vi "Build Help.vi"(8 "Error In":errorcluster) -> (0 "Error Out":errorcluster, 3 "stdout":string)   [LabVIEW 2017, in "Scripts.lvlib"]
uses:
  Scripts.lvlib
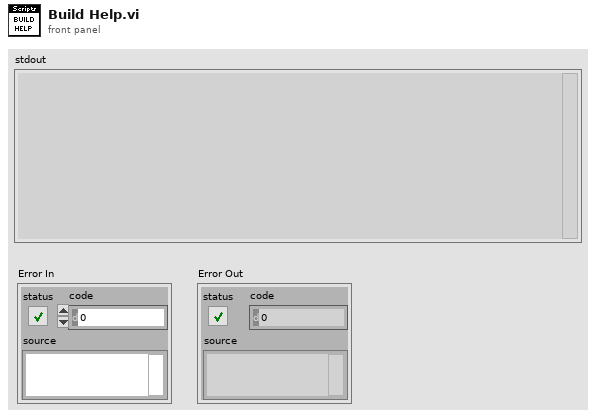
[diagram p1: front panel]
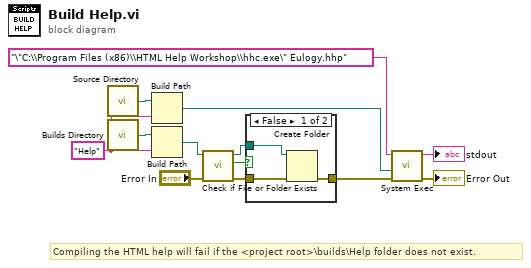
[diagram p0: block diagram]
diagram:
  w7 = "Help" ("name or relative path")
  # "Compiling the HTML help will fail if the <project root>\\builds\\Help folder does not exist."
  n1 = call "Source Directory.vi"() -> ("Source Directory"=w12:path)
  n2 = call "Builds Directory.vi"() -> ("Builds Directory"=w8:path)
  n3 = Build Path(base path=w12, name or relative path=w7) -> (appended path=w11:path)
  n4 = Build Path(base path=w8, name or relative path=w7) -> (appended path=w6:path)
  n5 = call <vilib>:"Check if File or Folder Exists.vi"("error in (no error)"="Error In", "path"=w6) -> ("error out"=w3:errorcluster, "file or folder exists?"=w4:bool, "dup path"=w1:path)  [unwired: 7 in]
  n6 = case shown="False" w4 {
    tunnel: w3 -> [w16 w17]
    tunnel: [w15 w17] -> w2
    tunnel: w1 -> [w14 _]
    frame False {
      n7 = Create Folder(path (use dialog)=w14, error in=w16) -> (error out=w15:errorcluster)  [unwired: 1 in, 2 out]
    }
    frame True {
    }
  }
  n8 = call <vilib>:"System Exec.vi"("error in (no error)"=w2, "working directory"=w11, "command line"="\"C:\\Program Files (x86)\\HTML Help Workshop\\hhc.exe\" Eulogy.hhp") -> ("error out"=→"Error Out":errorcluster, "standard output"=→"stdout":string)  [unwired: 5 in, 2 out]
